vi "PXI_acq.vi"(9 "O PXIs":T1[](array[typedef]), 10 "Sampels/Ch":i32, 11 "Tasks":refnum<k21>[](array[refnum])) -> (0 "Runs":u32[](array[numeric]), 1 "Indices":i32[][](array[numeric]), 3 "Data":dbl[][][](array[numeric]))   [LabVIEW 2013]
uses:
  AcqControls/Tasks_Indices.ctl
  <vilib>/DAQmx/read.llb/DAQmx Read (Analog 2D DBL NChan NSamp).vi
  <vilib>/DAQmx/miscellaneous.llb/DAQmx Fill In Error Info.vi
  <resource>/objmgr/daqmx.rc
panel:
  in  "PXI i":i32[][](array[numeric])
  out "CurrReadPos 2":dbl=1024.0
  out "AvailSampPerChan 2":u32
  out "TotalSampPerChanAcquired 2":dbl=1024.0
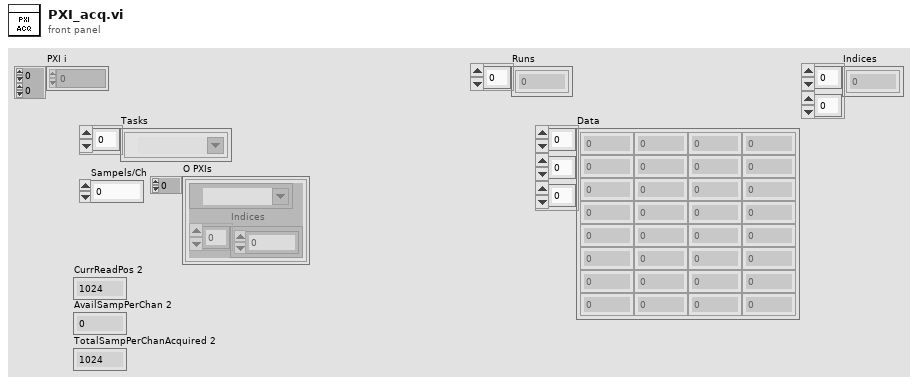
[diagram p1: front panel]
types:
  T1 = typedef "Tasks_Indices.ctl" = cluster{"task out":refnum<k21>, "Indices":i32[]}
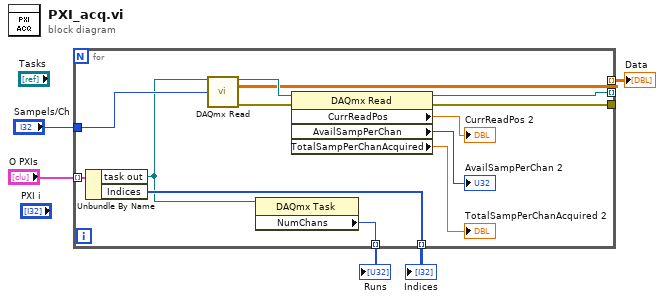
[diagram p0: block diagram]
diagram:
  n1 = for {
    tunnel: [w15] -> _ mode=indexing
    tunnel: [w12] -> _
    tunnel: "Sampels/Ch" -> [w11]
    tunnel: [w10] -> w4 mode=indexing
    tunnel: "O PXIs" -> [w9] mode=indexing
    tunnel: [w8] -> w2 mode=indexing
    tunnel: [w6] -> w1 mode=indexing
    n2 = Unbundle By Name(w9) -> ("task out"=w7:refnum<k21>, "Indices"=w8:i32[])
    n3 = call-poly <vilib>:"DAQmx Read.vi"("task/channels in"=w7, "number of samples per channel"=w11) -> ("task out"=w16:refnum<k21>, "data"=w10:dbl[][], "error out"=w13:errorcluster)  [unwired: 2 in, 9 out]
    n4 = property class="DAQmx Task"(reference=w7) -> ("NumChans"=w6:u32)  [unwired: 1 in, 2 out]
    n5 = property class="DAQmx Read"(reference=w16, error in=w13) -> (reference out=w15:refnum<k21>, error out=w12:errorcluster, "CurrReadPos"=→"CurrReadPos 2":dbl, "AvailSampPerChan"=→"AvailSampPerChan 2":u32, "TotalSampPerChanAcquired"=→"TotalSampPerChanAcquired 2":dbl)
  }
  "Data" <- w4
  "Indices" <- w2
  "Runs" <- w1
